vi "Calc Texel Starting Conditions.vi"(9 "Texture":T1, 10 "Flat Bottom Triangle":bool, 11 "UVs":cluster{"Top":T3, "Middle":T3, "Bottom":T3} {"Top"."v" min=0 max=1 step=0.1; "Top"."u" min=0 max=1 step=0.1; "Middle"."v" min=0 max=1 step=0.1; "Middle"."u" min=0 max=1 step=0.1; "Bottom"."v" min=0 max=1 step=0.1; "Bottom"."u" min=0 max=1 step=0.1}) -> (3 "Step Deltas (Texels Per Step)":T4 {"Texel Start"."v" min=0 max=1 step=0.1; "Texel Start"."u" min=0 max=1 step=0.1; "Texel End"."v" min=0 max=1 step=0.1; "Texel End"."u" min=0 max=1 step=0.1})   [LabVIEW 2022 SP3, in "Raster.lvlib"]
uses:
  Raster.lvlib
  Texel Step Deltas.ctl
  UV.ctl
  Rectangle Dimensions.ctl
  Texture.ctl
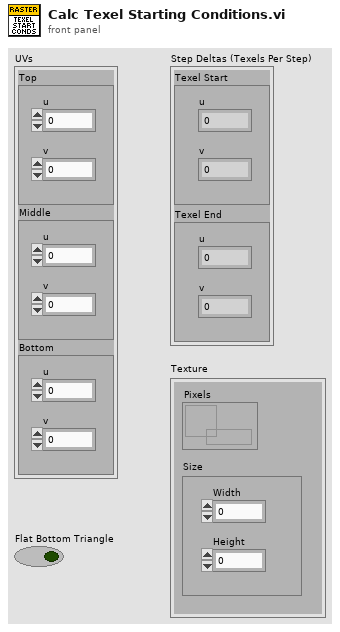
[diagram p1: front panel]
types:
  T1 = typedef "Raster.lvlib/Texture.ctl" = cluster{"Pixels":refnum<data-value>, "Size":T2}
  T2 = typedef "Raster.lvlib/Rectangle Dimensions.ctl" = cluster{"Width":u32, "Height":u32}
  T3 = typedef "Raster.lvlib/UV.ctl" = cluster{"u":sgl, "v":sgl}
  T4 = typedef "Raster.lvlib/Texel Step Deltas.ctl" = cluster{"Texel Start":T3, "Texel End":T3}
  T5 = typedef "Raster.lvlib/Point 2D.ctl" = cluster{"x":i32, "y":i32}
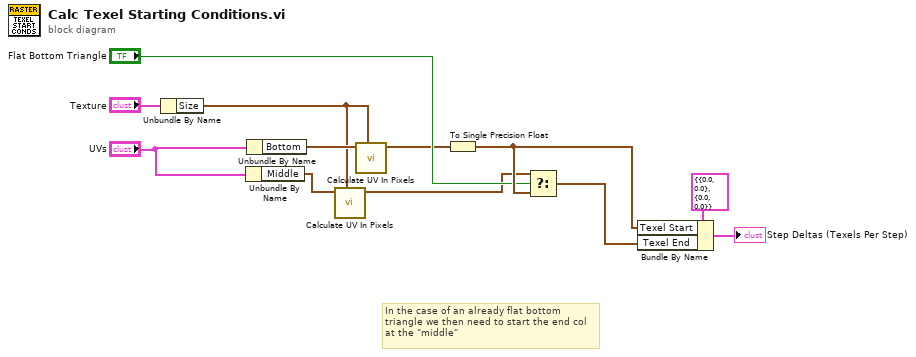
[diagram p0: block diagram]
diagram:
  # "In the case of an already flat bottom triangle we then need to start the end col at the \"middle\""
  n1 = Unbundle By Name("Texture") -> ("Size"=w1:T2)
  n2 = Unbundle By Name("UVs") -> ("Middle"=w6:T3)
  n3 = Unbundle By Name("UVs") -> ("Bottom"=w3:T3)
  n4 = call "Calculate UV In Pixels.vi"("Texture Dimensions"=w1, "UV"=w6) -> ("Pixels"=w7:T5)  [unwired: 9 in]
  n5 = call "Calculate UV In Pixels.vi"("Texture Dimensions"=w1, "UV"=w3) -> ("Pixels"=w4:T5)  [unwired: 9 in]
  n6 = To Single Precision Float(number=w4) -> (single precision float=w10:cluster{"x":sgl, "y":sgl})
  n7 = Select(t=w7, s="Flat Bottom Triangle", f=w10) -> (s? t:f=w12:cluster{"x":sgl, "y":sgl})
  n8 = Bundle By Name(cluster=T4 {"Texel Start"={"u"=0.0, "v"=0.0}, "Texel End"={"u"=0.0, "v"=0.0}} ("Step Deltas (Texels Per Step)"), "Texel Start"=w10, "Texel End"=w12) -> (→"Step Deltas (Texels Per Step)":T4)
